vi "configurePerChannel.vi"(8 "error in (no error)":errorcluster, 10 "physical channels":string, 11 "K2602 in":refnum<class "K2602.lvclass">) -> (0 "error out":errorcluster, 3 "K2602 out":refnum<class "K2602.lvclass">)   [LabVIEW 2011, in "Hardware.lvlib" / "Channels.lvlib" / "K2602.lvclass"]
uses:
  K2602.lvclass
  K2602.lvclass/K2602.ctl
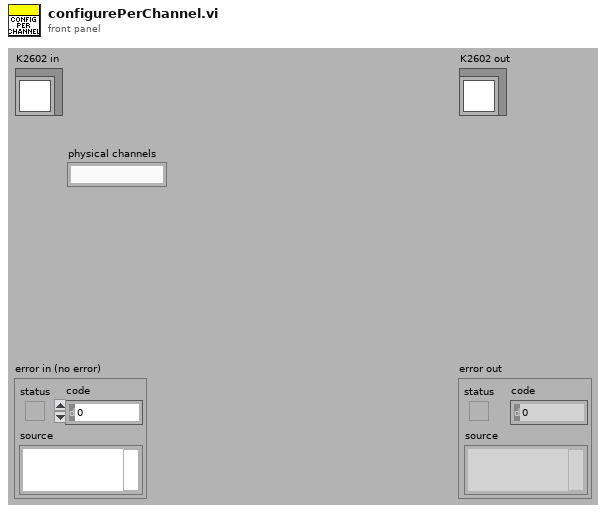
[diagram p1: front panel]
types:
  T1 = cluster{"Range":cluster{"current":dbl, "voltage":dbl}, "triggering_inUse":cluster{"start_trigger":string, "clock":string}, "Limits":cluster{"VoltageLimit":dbl, "CurrentLimit":dbl}}[]
  T2 = cluster{"Range":cluster{"current":dbl, "voltage":dbl}, "triggering_inUse":cluster{"start_trigger":string, "clock":string}, "Limits":cluster{"VoltageLimit":dbl, "CurrentLimit":dbl}}
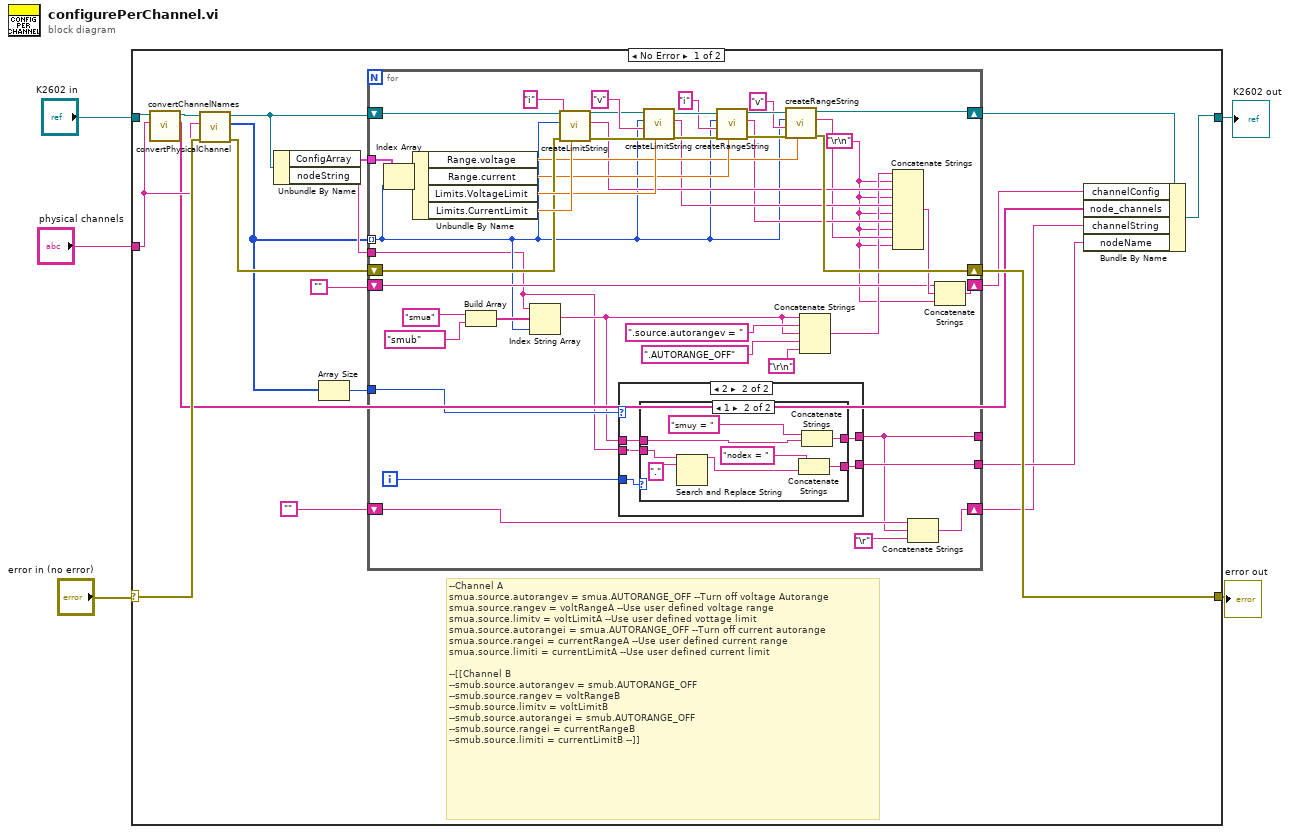
[diagram p0: block diagram]
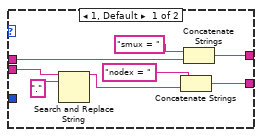
[diagram p2: hidden frame]
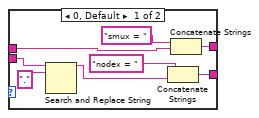
[diagram p3: hidden frame]
diagram:
  n1 = case shown="No Error" "error in (no error)" {
    selector: "error in (no error)" -> [w22 w99]
    tunnel: "K2602 in" -> [w14 w100]
    tunnel: [w18 w100] -> w3
    tunnel: [w24 w99] -> w2
    tunnel: "physical channels" -> [w13 _]
    frame No Error {
      # "--Channel A\nsmua.source.autorangev = smua.AUTORANGE_OFF --Turn off voltage Autorange\nsmua.source.rangev = voltRangeA --Use user defined voltage range\nsmua.source.limitv = voltLimitA --Use user defined vottage limit\nsmua.source.autorangei = smua.AUTORANGE_OFF --Turn off current autorange\nsmua.source.rangei = currentRangeA --Use user defined current range\nsmua.source.limiti = currentLimitA --Use user defined current limit\n\n--[[Channel B\n--smub.source.autorangev = smub.AUTORANGE_OFF\n--smub.source.rangev = voltRangeB\n--smub.source.limitv = voltLimitB\n--smub.source.autorangei = smub.AUTORANGE_OFF\n--smub.source.rangei = currentRangeB\n--smub.source.limiti = currentLimitB --]]"
      n2 = call "convertChannelNames.vi"("physicalChannels"=w13, "K2602 in"=w14) -> ("channels"=w12:string[], "K2602 out"=w15:refnum<class "K2602.lvclass">)  [unwired: 7 in, 1 out]
      n3 = call "convertPhysicalChannel.vi"("error in (no error)"=w22, "physicalChannels"=w13, "K2602 in"=w15) -> ("error out"=w23:errorcluster, "channel"=w10:i32[], "K2602 out"=w21:refnum<class "K2602.lvclass">)  [unwired: 6 in]
      n4 = Unbundle By Name(w21) -> ("ConfigArray"=w16:T1, "nodeString"=w17:string)
      n5 = Array Size(array=w10) -> (size(s)=w9:i32)
      n6 = for {
        shift-right: [w54] -> w19
        shift-left: w21 -> [w69]
        shift-right: [w52] -> w24
        shift-left: w23 -> [w62]
        tunnel: w10 -> [w35] mode=indexing
        shift-right: [w45] -> w11
        shift-left: "" -> [w46]
        tunnel: w17 -> [w31]
        tunnel: w16 -> [w36]
        tunnel: w9 -> [w33]
        tunnel: [w27] -> _
        tunnel: [w30] -> w8
        shift-right: [w25] -> w6
        shift-left: "" -> [w28]
        i -> [w29]
        w39 = "\r\n"
        n7 = Index Array(array=w36, index=w35) -> (element=w34:T2)
        n8 = Unbundle By Name(w34) -> ("Range.voltage"=w53:dbl, "Range.current"=w58:dbl, "Limits.VoltageLimit"=w63:dbl, "Limits.CurrentLimit"=w64:dbl)
        n9 = Build Array("smua", "smub") -> (w42:string[])
        n10 = Index String Array(1:w35, 2:w42, 3:w31) -> (0:w32:string)
        n11 = call "createLimitString.vi"("Limit (0.000)"=w64, "error in (no error)"=w62, "Function"="i", "Channel (Channel A)"=w35, "K2602 in"=w69) -> ("error out"=w65:errorcluster, "Limit string"=w51:string, "K2602 out"=w66:refnum<class "K2602.lvclass">)  [unwired: 4 in]
        n12 = case shown="2" w33 {
          tunnel: w32 -> [w76 w81]
          tunnel: w31 -> [w72 w80]
          tunnel: [w74 w79] -> w27
          tunnel: [w73 w78] -> w30
          tunnel: w29 -> [_ w82]
          frame 1, Default {
            n13 = Search and Replace String(input string=w72, search string=".") -> (result string=w70:string)  [unwired: 6 in, 3 out]
            n14 = Concatenate Strings("nodex = ", w70) -> (w73:string)
            n15 = Concatenate Strings("smux = ", w76) -> (w74:string)
          }
          frame 2 {
            n16 = case shown="1" w82 {
              tunnel: w81 -> [w86 w94]
              tunnel: w80 -> [w85 w93]
              tunnel: [w84 w92] -> w79
              tunnel: [w83 w91] -> w78
              frame 0, Default {
                n17 = Search and Replace String(input string=w85, search string=".") -> (result string=w87:string)  [unwired: 6 in, 3 out]
                n18 = Concatenate Strings("nodex = ", w87) -> (w83:string)
                n19 = Concatenate Strings("smux = ", w86) -> (w84:string)
              }
              frame 1 {
                n20 = Search and Replace String(input string=w93, search string=".") -> (result string=w95:string)  [unwired: 6 in, 3 out]
                n21 = Concatenate Strings("nodex = ", w95) -> (w91:string)
                n22 = Concatenate Strings("smuy = ", w94) -> (w92:string)
              }
            }
          }
        }
        n23 = call "createLimitString.vi"("Limit (0.000)"=w63, "error in (no error)"=w65, "Function"="v", "Channel (Channel A)"=w35, "K2602 in"=w66) -> ("error out"=w61:errorcluster, "Limit string"=w50:string, "K2602 out"=w60:refnum<class "K2602.lvclass">)  [unwired: 4 in]
        n24 = call "createRangeString.vi"("range (0.000)"=w58, "error in (no error)"=w61, "Function"="i", "Channel (Channel A)"=w35, "K2602 in"=w60) -> ("error out"=w57:errorcluster, "Limit string"=w49:string, "K2602 out"=w56:refnum<class "K2602.lvclass">)  [unwired: 4 in]
        n25 = call "createRangeString.vi"("range (0.000)"=w53, "error in (no error)"=w57, "Function"="v", "Channel (Channel A)"=w35, "K2602 in"=w56) -> ("error out"=w52:errorcluster, "Limit string"=w48:string, "K2602 out"=w54:refnum<class "K2602.lvclass">)  [unwired: 4 in]
        n26 = Concatenate Strings(w32, ".source.autorangev = ", w32, ".AUTORANGE_OFF", "\r\n") -> (w40:string)
        n27 = Concatenate Strings(w40, w39, w51, w39, w50, w39, w49, w39, w48, w39) -> (w47:string)
        n28 = Concatenate Strings(w28, w27, "\r") -> (w25:string)
        n29 = Concatenate Strings(w46, w47, w39) -> (w45:string)
      }
      n30 = Bundle By Name(cluster=w19, "channelConfig"=w11, "node_channels"=w12, "channelString"=w6, "nodeName"=w8) -> (w18:refnum<class "K2602.lvclass">)
    }
    frame Error {
    }
  }
  "error out" <- w2
  "K2602 out" <- w3
